vi "MenuItem (SubVI).vi"(6 "UserEvent In":refnum<user-event>, 7 "MenuItem":T2, 8 "error in (no error)":errorcluster, 9 "Account":string, 10 "UserInputState":T1=enum."Deposit", 11 "Display Queue in":refnum<queue>) -> (0 "error out":errorcluster, 2 "UserInputState 2":T1, 3 "Display Queue out":refnum<queue>)   [LabVIEW 2017]
doc: "This VI performs functions depending on the Menu Item selected. The User Input state is determined by this VI to be used."
uses:
  Controls/DisplayControl.ctl
  Controls/DisplayCommand.ctl
  Controls/MenuItem.ctl
  Controls/UserInputState.ctl
  Controls/EnableDisableCommand.ctl
  Controls/UpdateMessageControl.ctl
  Controls/UpdateMessageCommand.ctl
  Global 2.vi
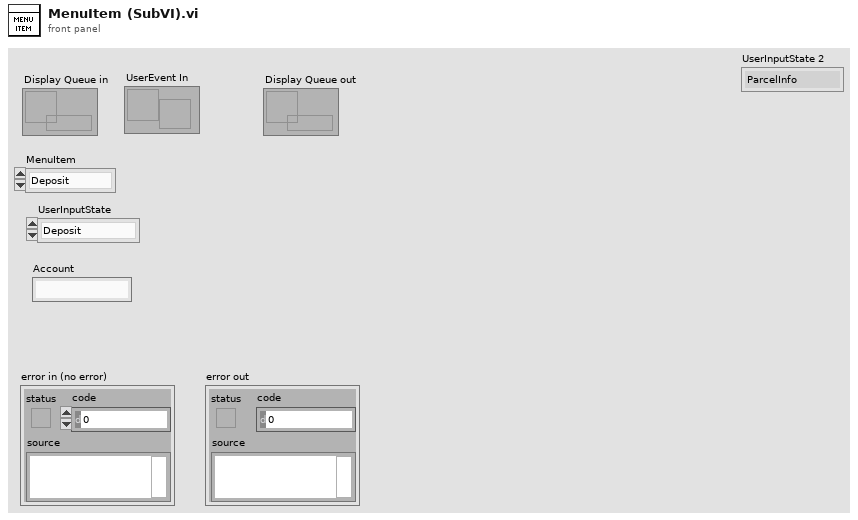
[diagram p1: front panel]
types:
  T1 = typedef "UserInputState.ctl" = enum16{"ParcelInfo", "PhoneInfo", "Deposit", "Withdrawal"}
  T2 = typedef "MenuItem.ctl" = enum16{"Deposit", "Finish", "Withdraw", "None"}
  T3 = typedef "UpdateMessageControl.ctl" = cluster{"Command":T4, "Data":variant}
  T4 = typedef "UpdateMessageCommand.ctl" = enum16{"Welcome", "MainMenu", "PhoneNumberFailed", "PhoneNumberSuccess", "ParcelNumberSuccess", "ParcelNumbertFailed", "SessionTerminate", "SessionFinished", "Deposit", "DepositComplete", "Withdrawal", "WithdrawalComplete", "WithdrawalFailed"}
  T5 = typedef "DisplayControl.ctl" = cluster{"Command":T6, "Data":variant}
  T6 = typedef "DisplayCommand.ctl" = enum16{"Initialize", "Open/Close Parcel", "Enable/Disable Controls", "FocusCursor", "UpdateMessage", "UpdateMenus", "FinishOperation", "Exit", "CleanUserInput"}
  T7 = typedef "EnableDisableCommand.ctl" = enum16{"InitialSetup", "EnableUserInput", "DisableUserInput", "EnableMenus", "DisableMenus"}
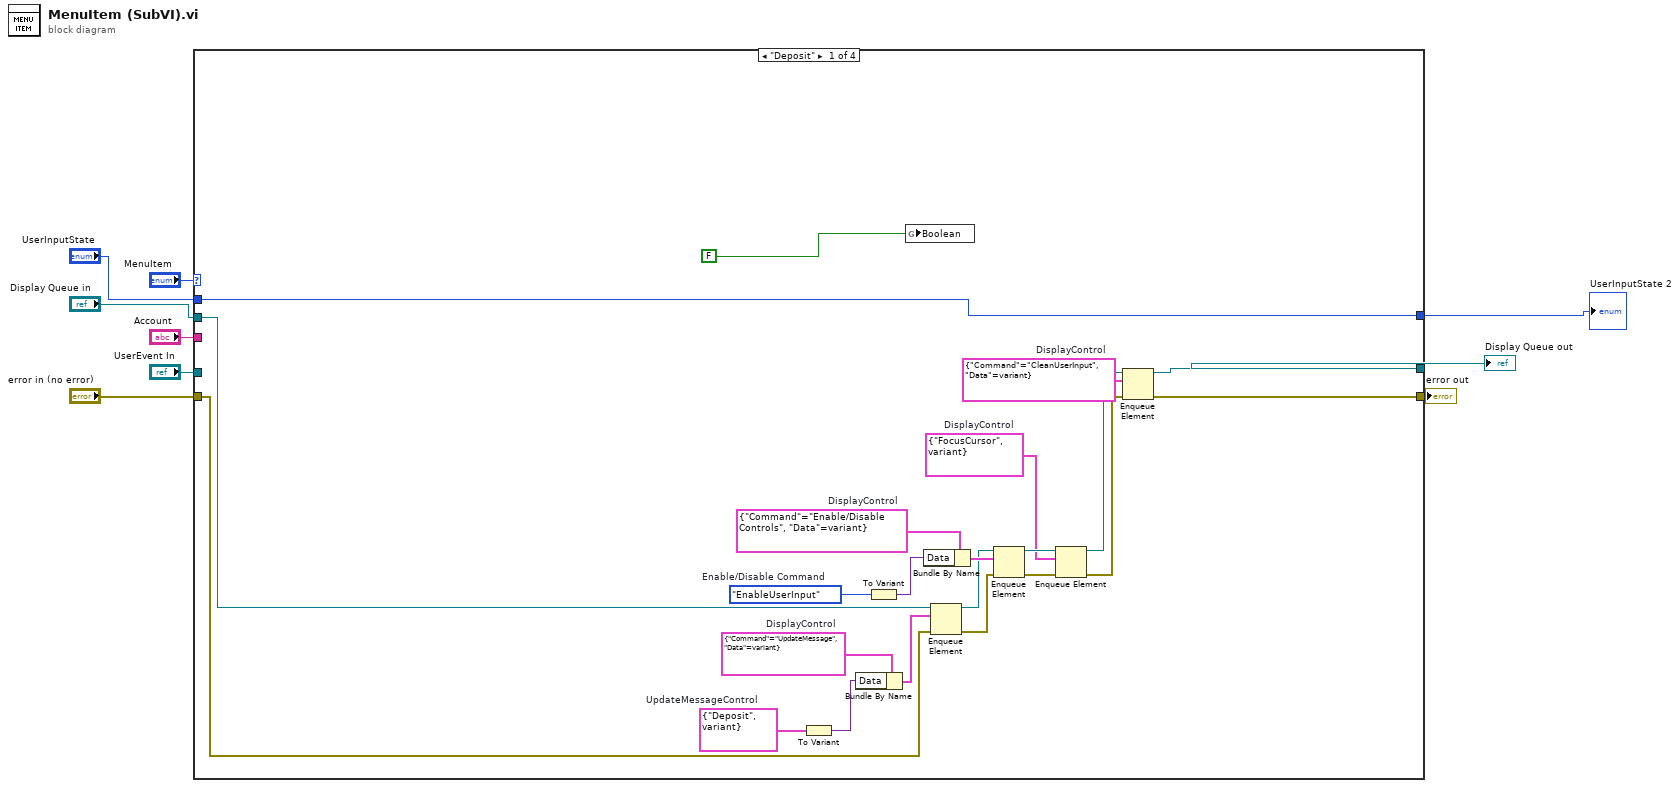
[diagram p0: block diagram]
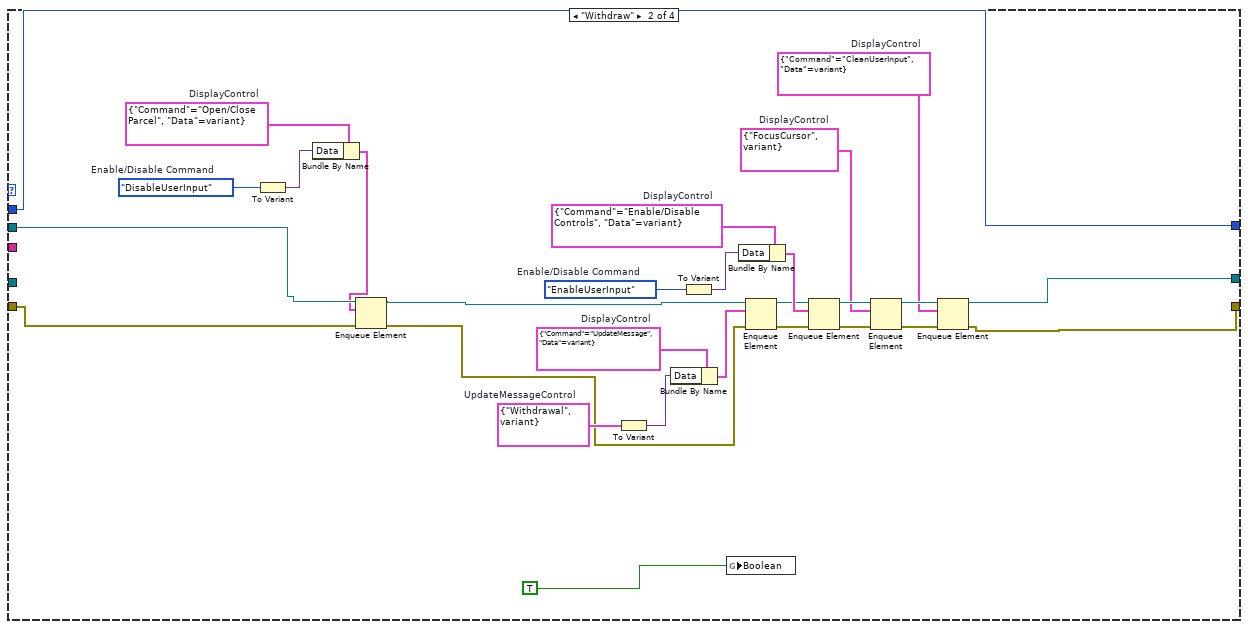
[diagram p2: hidden frame]
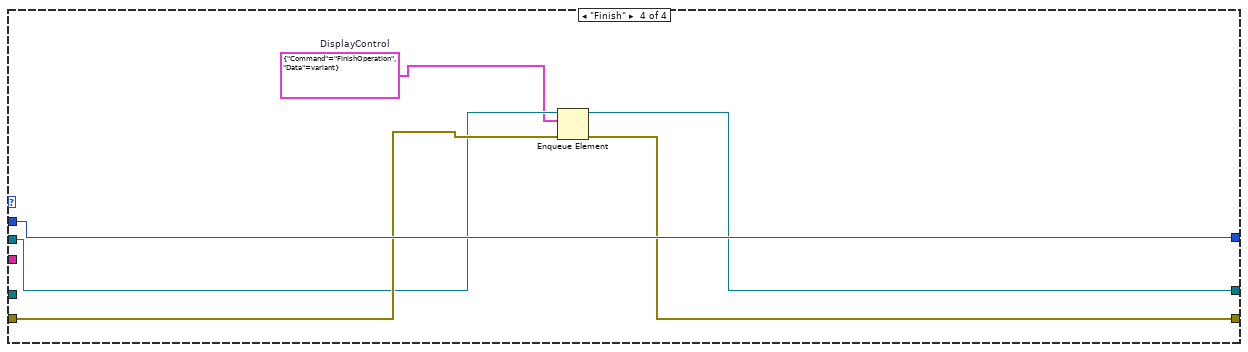
[diagram p4: hidden frame]
diagram:
  n1 = case shown="\"Deposit\"" "MenuItem" {
    tunnel: "Display Queue in" -> [w15 w38 w61 w65]
    tunnel: "error in (no error)" -> [w14 w40 w62 w67]
    tunnel: [w20 w42 w62 w66] -> w7
    tunnel: [w21 w41 w61 w64] -> w6
    tunnel: [w11 w43 w60 w68] -> w1
    tunnel: "Account" -> [_ _ _ _]
    tunnel: "UserInputState" -> [w11 w43 w60 w68]
    tunnel: "UserEvent In" -> [_ _ _ _]
    frame "Deposit" {
      w12 = T3 {"Command"=enum."Deposit", "Data"=variant}  # UpdateMessageControl
      w19 = T5 {"Command"=enum."UpdateMessage", "Data"=variant}  # DisplayControl
      w22 = T5 {"Command"=enum."CleanUserInput", "Data"=variant}  # DisplayControl
      w25 = T5 {"Command"=enum."FocusCursor", "Data"=variant}  # DisplayControl
      w30 = EnableDisableCommand."EnableUserInput"  # Enable/Disable Command
      w28 = T5 {"Command"=enum."Enable/Disable Controls", "Data"=variant}  # DisplayControl
      n2 = To Variant(anything=w12) -> (Variant=w17:variant)
      n3 = Bundle By Name(cluster=w19, "Data"=w17) -> (w18:T5)
      n4 = To Variant(anything=w30) -> (Variant=w31:variant)
      n5 = global write "Global 2.vi" "Boolean"(FALSE) -> ()
      n6 = Bundle By Name(cluster=w28, "Data"=w31) -> (w29:T5)
      n7 = Enqueue Element(queue=w15, element=w18, error in (no error)=w14) -> (queue out=w16:refnum<queue>, error out=w13:errorcluster)  [unwired: 1 in, 1 out]
      n8 = Enqueue Element(queue=w16, element=w29, error in (no error)=w13) -> (queue out=w27:refnum<queue>, error out=w26:errorcluster)  [unwired: 1 in, 1 out]
      n9 = Enqueue Element(queue=w27, element=w25, error in (no error)=w26) -> (queue out=w24:refnum<queue>, error out=w23:errorcluster)  [unwired: 1 in, 1 out]
      n10 = Enqueue Element(queue=w24, element=w22, error in (no error)=w23) -> (queue out=w21:refnum<queue>, error out=w20:errorcluster)  [unwired: 1 in, 1 out]
    }
    frame "Withdraw" {
      w33 = EnableDisableCommand."DisableUserInput"  # Enable/Disable Command
      w36 = T5 {"Command"=enum."Open/Close Parcel", "Data"=variant}  # DisplayControl
      w44 = T3 {"Command"=enum."Withdrawal", "Data"=variant}  # UpdateMessageControl
      w47 = T5 {"Command"=enum."UpdateMessage", "Data"=variant}  # DisplayControl
      w50 = T5 {"Command"=enum."CleanUserInput", "Data"=variant}  # DisplayControl
      w53 = T5 {"Command"=enum."FocusCursor", "Data"=variant}  # DisplayControl
      w58 = EnableDisableCommand."EnableUserInput"  # Enable/Disable Command
      w56 = T5 {"Command"=enum."Enable/Disable Controls", "Data"=variant}  # DisplayControl
      n11 = To Variant(anything=w33) -> (Variant=w34:variant)
      n12 = Bundle By Name(cluster=w36, "Data"=w34) -> (w35:T5)
      n13 = Enqueue Element(queue=w38, element=w35, error in (no error)=w40) -> (queue out=w37:refnum<queue>, error out=w39:errorcluster)  [unwired: 1 in, 1 out]
      n14 = To Variant(anything=w44) -> (Variant=w49:variant)
      n15 = Bundle By Name(cluster=w47, "Data"=w49) -> (w48:T5)
      n16 = To Variant(anything=w58) -> (Variant=w59:variant)
      n17 = global write "Global 2.vi" "Boolean"(TRUE) -> ()
      n18 = Bundle By Name(cluster=w56, "Data"=w59) -> (w57:T5)
      n19 = Enqueue Element(queue=w37, element=w48, error in (no error)=w39) -> (queue out=w45:refnum<queue>, error out=w46:errorcluster)  [unwired: 1 in, 1 out]
      n20 = Enqueue Element(queue=w45, element=w57, error in (no error)=w46) -> (queue out=w55:refnum<queue>, error out=w54:errorcluster)  [unwired: 1 in, 1 out]
      n21 = Enqueue Element(queue=w55, element=w53, error in (no error)=w54) -> (queue out=w52:refnum<queue>, error out=w51:errorcluster)  [unwired: 1 in, 1 out]
      n22 = Enqueue Element(queue=w52, element=w50, error in (no error)=w51) -> (queue out=w41:refnum<queue>, error out=w42:errorcluster)  [unwired: 1 in, 1 out]
    }
    frame "None", Default {
      # "This case can be used for future ATM functions"
    }
    frame "Finish" {
      w63 = T5 {"Command"=enum."FinishOperation", "Data"=variant}  # DisplayControl
      n23 = Enqueue Element(queue=w65, element=w63, error in (no error)=w67) -> (queue out=w64:refnum<queue>, error out=w66:errorcluster)  [unwired: 1 in, 1 out]
    }
  }
  "error out" <- w7
  "Display Queue out" <- w6
  "UserInputState 2" <- w1
